vi "Read thickness from DB.vi"(8 "error in (no error)":errorcluster, 10 "Module?":bool, 11 "Database Entry in":refnum<class "Database Entry.lvclass">) -> (0 "error out":errorcluster, 1 "Baselayer IDs":string[](array[string]), 2 "DB out baselayer":string[][](array[string]), 3 "Database Entry out":refnum<class "Database Entry.lvclass">, 4 "Replace parts":bool, 5 "Stack names":string[](array[string]))   [LabVIEW 2021, in "Database Entry.lvclass"]
uses:
  Database Entry.lvclass
  Database Entry.lvclass/Database Entry.ctl
  <vilib>/Utility/file.llb/Read Delimited Spreadsheet (string).vi
  Components/Stack/Stack.lvclass
panel:
  out "DB out stack":string[][](array[string])
  out "DB out toplayer":string[][](array[string])
  out "Toplayer IDs":string[](array[string])
  out "error out py":errorcluster
  in  "error in (no error) py":errorcluster
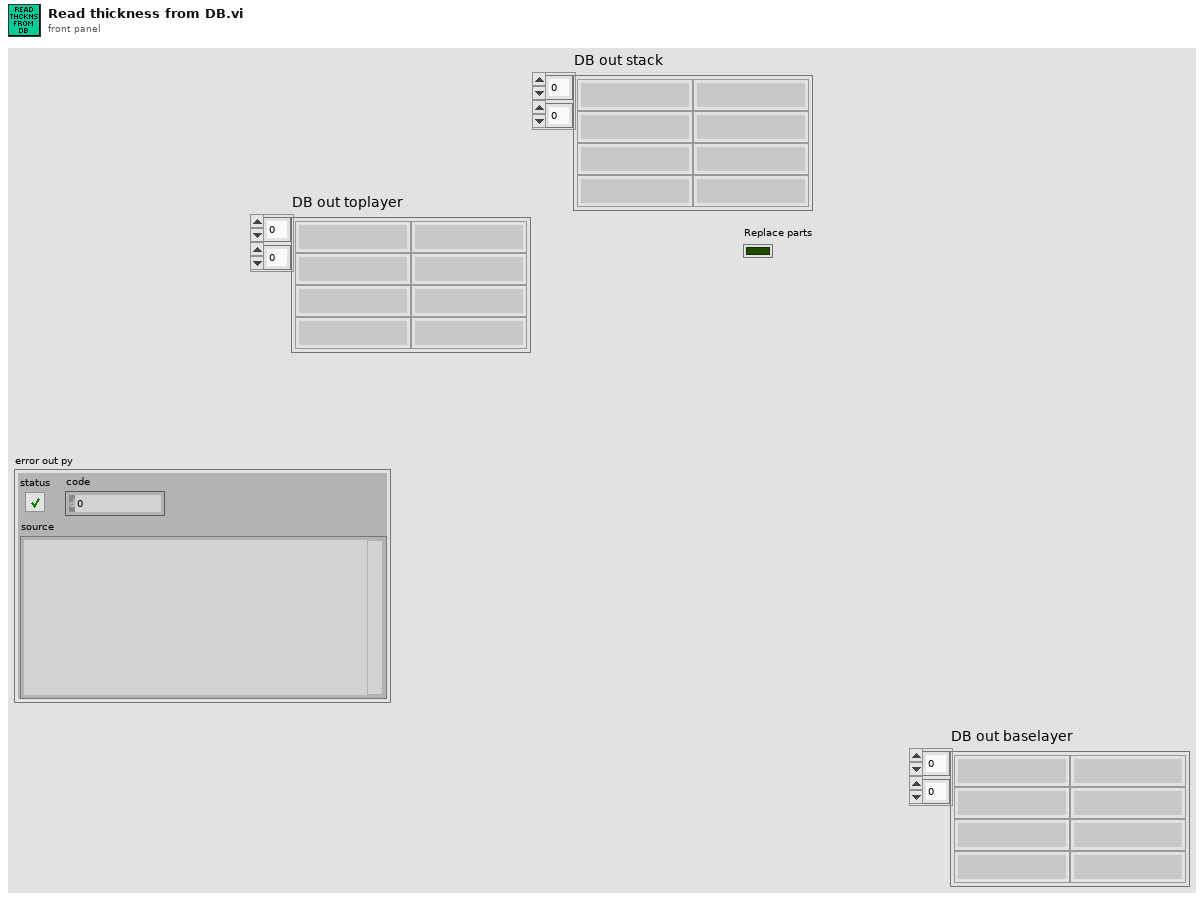
[diagram p1: front panel]
types:
  T1 = cluster{"type (proto/module)":string, " geometry":string, "resolution":string, "baselayer":string, "toplayer":string, "bl_pos":string, "tl_pos":string, "put_pos":string, "region":string, "asstray":string, "comptray":string, "put":string, "date":string, "timestart":string, "timeend":string, "operator":string, "tape":string, "glue":string, "stack name":string, "Adhesive type":string, "Comments":string, "Temperature":string, "Relative Humidity":string, "Sensor grade":string, "ROC version":string, "Baseplate material":string}
  T2 = typedef "File Paths.ctl" = cluster{"Glue Pattern Folder":path, "Carrier Tray Folder":path, "Pick Up Tool Fixture Folder":path, "Components Folder":path, "Bellows Tool Offset.txt":path, "Pick Up Tool Offset.txt":path, "Dispense Tip Offset.txt":path, "Log Files":path, "Gantry Assembly Map.txt":path, "Syringe and offset map.txt":path, "Controllers Folder":path, "Local dbase config":path}
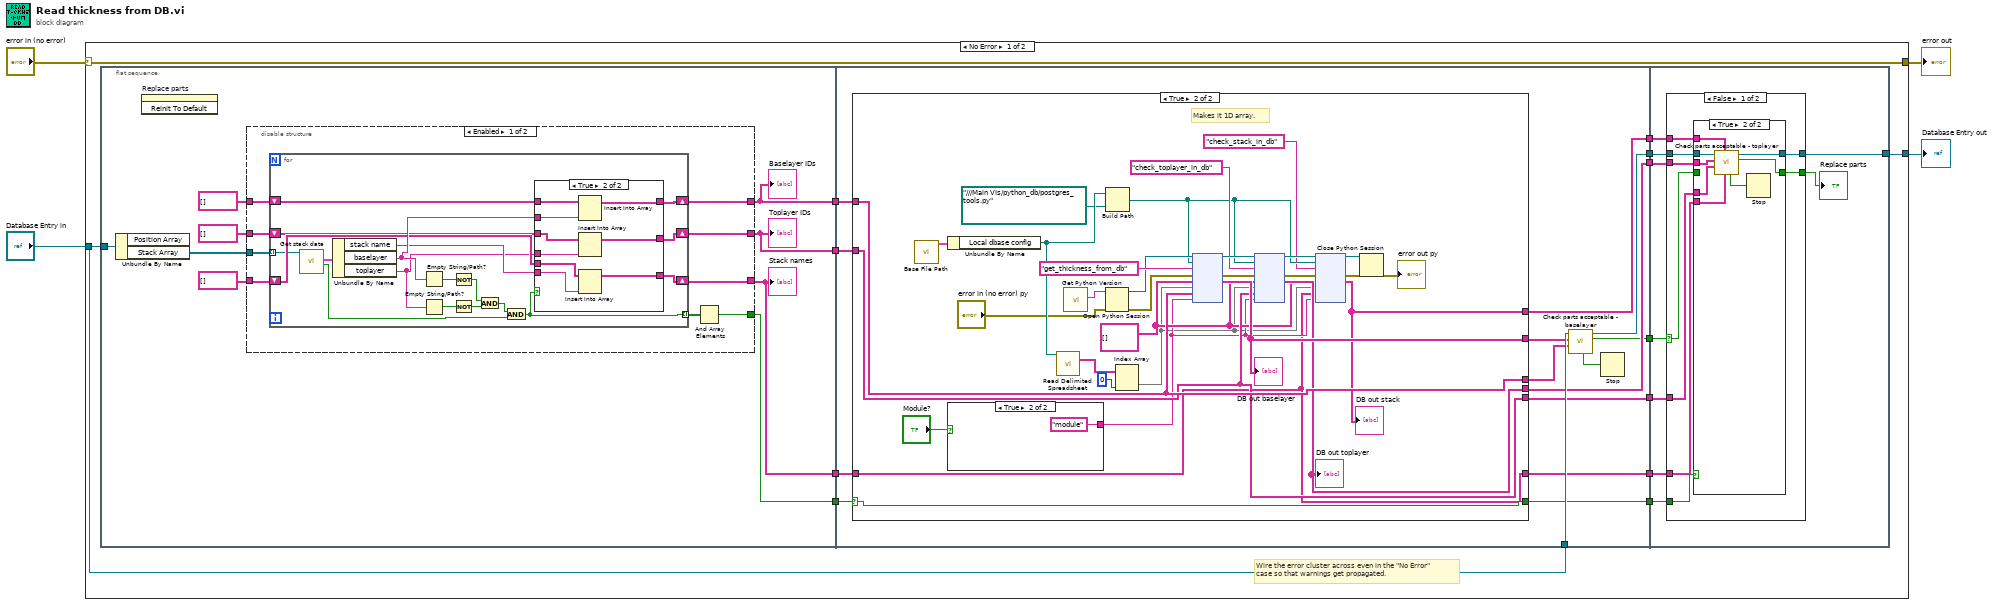
[diagram p0: block diagram]
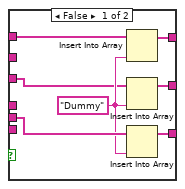
[diagram p2: hidden frame]
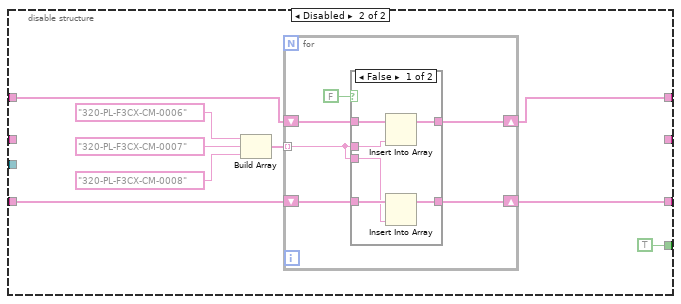
[diagram p3: hidden frame]
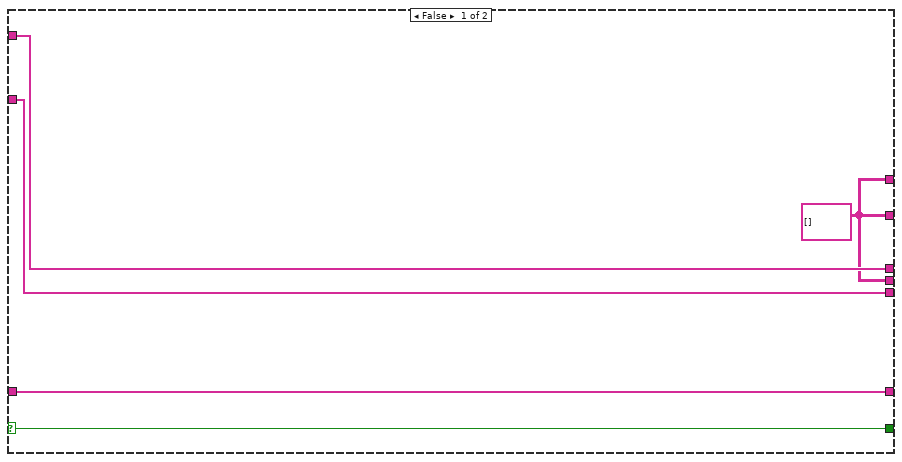
[diagram p5: hidden frame]
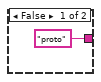
[diagram p6: hidden frame]
diagram:
  n1 = case shown="No Error" "error in (no error)" {
    selector: "error in (no error)" -> [w18 w178]
    tunnel: [w18 w178] -> w3
    tunnel: [w14 w177] -> w1
    tunnel: "Database Entry in" -> [w15 w177]
    frame No Error {
      # "Wire the error cluster across even in the \"No Error\"\ncase so that warnings get propagated."
      n2 = flat-sequence {
        tunnel: [w25] -> w17
        tunnel: [w22] -> w16
        tunnel: w15 -> [w27]
        tunnel: [w20] -> w13
        tunnel: [w19] -> w7
        tunnel: w17 -> [w108]
        tunnel: w16 -> [w107]
        tunnel: w15 -> [w106]
        tunnel: w13 -> [w101]
        tunnel: [w104] -> w12
        tunnel: [w100] -> w11
        tunnel: [w99] -> w10
        tunnel: [w98] -> w9
        tunnel: [w97] -> w8
        tunnel: w7 -> [w96]
        tunnel: [w95] -> w6
        tunnel: [w94] -> w5
        tunnel: [w154] -> w14
        tunnel: w12 -> [w155]
        tunnel: w11 -> [w153]
        tunnel: w10 -> [w152]
        tunnel: w9 -> [w151]
        tunnel: w8 -> [w149]
        tunnel: w6 -> [w148]
        tunnel: w5 -> [w147]
        frame #0 {
          n3 = Unbundle By Name(w27) -> ("Stack Array"=w26:refnum<class "Stack.lvclass">[])  [unwired: 1 out]
          n4 = invoke on="Replace parts" class="Bool (strict)" method="Reinit To Default"() -> ()  [unwired: 3 in, 3 out]
          n5 = disable-structure shown="Enabled" {
            disable-tunnel: w26 -> [w36 _]
            disable-tunnel: [w35 w79] -> w25
            disable-tunnel: string[] [] -> [w34 w77]
            disable-tunnel: string[] [] -> [w33 w76]
            disable-tunnel: [w32 w78] -> w19
            disable-tunnel: [w30 TRUE] -> w22
            disable-tunnel: [w28 _] -> w20
            disable-tunnel: string[] [] -> [w29 _]
            frame Enabled {
              n6 = for {
                tunnel: w36 -> [w48] mode=indexing
                shift-right: [w53] -> w35
                shift-left: w34 -> [w54]
                shift-right: [w50] -> w32
                shift-left: w33 -> [w51]
                tunnel: [w40] -> w31 mode=indexing
                shift-right: [w37] -> w28
                shift-left: w29 -> [w39]
                n7 = call "Get stack data.vi"("Stack in"=w48) -> ("Is real run"=w46:bool, "Data cluster"=w47:T1)  [unwired: 7 in, 2 out]
                n8 = Unbundle By Name(w47) -> ("stack name"=w49:string, "baselayer"=w52:string, "toplayer"=w38:string)
                n9 = Empty String/Path?(string/path=w52) -> (empty?=w45:bool)
                n10 = Empty String/Path?(string/path=w38) -> (empty?=w44:bool)
                n11 = Not(x=w45) -> (.not. x?=w43:bool)
                n12 = Not(x=w44) -> (.not. x?=w42:bool)
                n13 = And(x=w43, y=w42) -> (x .and. y?=w41:bool)
                n14 = And(x=w41, y=w46) -> (x .and. y?=w40:bool)
                n15 = case shown="True" w40 {
                  tunnel: w54 -> [w61 w70]
                  tunnel: [w60 w69] -> w53
                  tunnel: w52 -> [_ w68]
                  tunnel: w51 -> [w59 w67]
                  tunnel: [w58 w66] -> w50
                  tunnel: w49 -> [_ w65]
                  tunnel: [w56 w64] -> w37
                  tunnel: w39 -> [w55 w63]
                  tunnel: w38 -> [_ w62]
                  frame False {
                    w57 = "Dummy" ("new element/subarray")
                    n16 = Insert Into Array(array=w61, new element=w57) -> (w60:string[])  [unwired: 1 in]
                    n17 = Insert Into Array(array=w55, new element=w57) -> (w56:string[])  [unwired: 1 in]
                    n18 = Insert Into Array(array=w59, new element=w57) -> (w58:string[])  [unwired: 1 in]
                  }
                  frame True {
                    n19 = Insert Into Array(array=w70, new element=w68) -> (w69:string[])  [unwired: 1 in]
                    n20 = Insert Into Array(array=w63, new element=w62) -> (w64:string[])  [unwired: 1 in]
                    n21 = Insert Into Array(array=w67, new element=w65) -> (w66:string[])  [unwired: 1 in]
                  }
                }
              }
              n22 = And Array Elements(Boolean array=w31) -> (logical AND=w30:bool)
            }
            frame Disabled {
              n23 = Build Array("320-PL-F3CX-CM-0006", "320-PL-F3CX-CM-0007", "320-PL-F3CX-CM-0008") -> (w71:string[])
              n24 = for {
                shift-right: [w85] -> w78
                shift-left: w76 -> [w80]
                shift-right: [w84] -> w79
                shift-left: w77 -> [w81]
                tunnel: w71 -> [w82] mode=indexing
                n25 = case shown="False" FALSE {
                  tunnel: w80 -> [w91 w93]
                  tunnel: [w90 w93] -> w85
                  tunnel: w82 -> [w89 _]
                  tunnel: w81 -> [w88 w92]
                  tunnel: w82 -> [w87 _]
                  tunnel: [w86 w92] -> w84
                  frame False {
                    n26 = Insert Into Array(array=w88, new element=w87) -> (w86:string[])  [unwired: 1 in]
                    n27 = Insert Into Array(array=w91, new element=w89) -> (w90:string[])  [unwired: 1 in]
                  }
                  frame True {
                  }
                }
              }
            }
          }
          "Baselayer IDs" <- w25
          "Stack names" <- w19
          "Toplayer IDs" <- w20
        }
        frame #1 {
          n28 = case shown="True" w107 {
            selector: w107 -> [w111 w125]
            tunnel: w108 -> [w113 w132]
            tunnel: [w110 w133] -> w105
            tunnel: [w113 w132] -> w103
            tunnel: w101 -> [w112 w126]
            tunnel: [w110 w127] -> w100
            tunnel: [w112 w126] -> w99
            tunnel: [w111 w125] -> w97
            tunnel: w96 -> [w109 w114]
            tunnel: [w110 w115] -> w95
            tunnel: [w109 w114] -> w94
            frame False {
              w110 = string[][] []
            }
            frame True {
              w120 = string[][] []
              # "Makes it 1D array."
              n29 = call "Base File Path.vi"() -> ("Paths Out"=w139:T2)  [unwired: 11 in]
              n30 = Unbundle By Name(w139) -> ("Local dbase config"=w142:path)
              n31 = case shown="True" "Module?" {
                tunnel: ["proto" "module"] -> w117
                frame False {
                }
                frame True {
                }
              }
              n32 = call-poly <vilib>:"Read Delimited Spreadsheet.vi"("file path (dialog if empty)"=w142) -> ("all rows"=w138:string[][])  [unwired: 9 in, 5 out]
              n33 = call "Get Python Version.vi"() -> ("Python Version"=w137:string)  [unwired: 10 in, 1 out]
              n34 = Open Python Session(python version=w137, 3:"error in (no error) py") -> (session out=w131:refnum<k35>, error out=w134:errorcluster)  [unwired: 1 in]
              n35 = Build Path(base path=w142, name or relative path=path "../../../Main VIs/python_db/postgres_tools.py" ("module path")) -> (appended path=w119:path)
              n36 = Index Array(array=w138, index (col)=0 ("disabled index (col)")) -> (element=w116:string[])  [unwired: 1 in]
              n37 = node(w131, w119, "get_thickness_from_db" ("function name"), w134, w120, w116, w132, w117) -> (w130:refnum<k35>, w128:errorcluster, w133:string[][])  [unwired: 3 in, 2 out]
              "DB out baselayer" <- w133
              n38 = node(w130, w119, "check_toplayer_in_db" ("function name"), w128, w120, w116, w126, w117) -> (w122:refnum<k35>, w124:errorcluster, w127:string[][])  [unwired: 3 in, 2 out]
              "DB out toplayer" <- w127
              n39 = node(w122, w119, "check_stack_in_db" ("function name"), w124, w120, w116, w114, w117) -> (w121:refnum<k35>, w123:errorcluster, w115:string[][])  [unwired: 3 in, 2 out]
              "DB out stack" <- w115
              n40 = Close Python Session(session in=w121, error in=w123) -> (11:→"error out py":errorcluster)
            }
          }
          n41 = call "Check parts acceptable - baselayer.vi"("Baselayer IDs"=w103, "DB out base"=w105, "Database Entry in"=w106) -> ("Replace parts out"=w98:bool, "Database Entry out"=w104:refnum<class "Database Entry.lvclass">, "Abort?"=w102:bool)  [unwired: 4 in, 2 out]
          n42 = Stop(stop? (T)=w102) -> ()
        }
        frame #2 {
          n43 = case shown="False" w151 {
            selector: w151 -> [w158 w175]
            tunnel: w155 -> [w164 w176]
            tunnel: [w163 w176] -> w154
            tunnel: w153 -> [w162 _]
            tunnel: w152 -> [w161 _]
            tunnel: [w160 w175] -> w150
            tunnel: w149 -> [w159 _]
            tunnel: w148 -> [w157 _]
            tunnel: w147 -> [w156 _]
            frame False {
              n44 = case shown="True" w159 {
                tunnel: w164 -> [w166 w174]
                tunnel: [w166 w173] -> w163
                tunnel: w162 -> [_ w172]
                tunnel: w161 -> [_ w171]
                tunnel: [w165 w169] -> w160
                tunnel: w158 -> [w165 _]
                tunnel: w157 -> [_ w168]
                tunnel: w156 -> [_ w167]
                frame False {
                }
                frame True {
                  n45 = call "Check parts acceptable - toplayer.vi"("Stack IDs"=w167, "DB out stack"=w168, "Toplayer IDs"=w171, "DB out top"=w172, "Database Entry in"=w174) -> ("Replace parts out"=w169:bool, "Database Entry out"=w173:refnum<class "Database Entry.lvclass">, "Abort?"=w170:bool)  [unwired: 3 in, 1 out]
                  n46 = Stop(stop? (T)=w170) -> ()
                }
              }
            }
            frame True {
            }
          }
          "Replace parts" <- w150
        }
      }
    }
    frame Error {
    }
  }
  "error out" <- w3
  "Database Entry out" <- w1
